vi "Fetch Measurement.vi"(6 "Enable Relative Mode (F: Disable)":bool, 7 "Combination (0: Single)":dbl(ring) items=["Single", "Feed1-Feed2", "Feed1/Feed2"], 8 "error in (no error)":errorcluster, 9 "Measurement Number (0: <0>)":i32(ring) items=["Measurement 1"=1, "Measurement 2"=2, "Measurement 3"=3, "Measurement 4"=4], 10 "Maximum Time (30000 ms)":dbl=30000.0, 11 "VISA resource name":refnum<visa-resource-name>) -> (0 "error out":errorcluster, 2 "Measurement Data (dBm or Volt)":dbl, 3 "VISA resource name out":refnum<visa-resource-name>)   [LabVIEW 2011, in "Agilent N432A.lvlib"]
doc: "Fetches the measurement data depending on the combination and relative mode settings. The combination parameter must be the same as that configured in the Configure Measurement.vi and the relative mode parameter must be the same as that configured in the Configure Relative Measurement.vi. You need to initiate an acquisition with the Initiate VI prior to calling this VI.\n\n<B>Note:</B>\n\nYou must use the Configure Measurement.vi and Configure Relative Measurement.vi to set the power meter before using this VI to fetch data.\n\nUse this VI only with other low-level VIs. The high-level VIs automatically incorporate this functionality. This VI does not check the instrument status."
uses:
  <instrlib>/Agilent N432A/Agilent N432A.lvlib
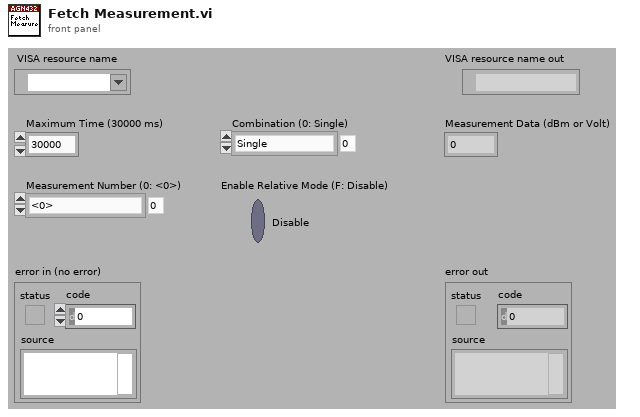
[diagram p1: front panel]
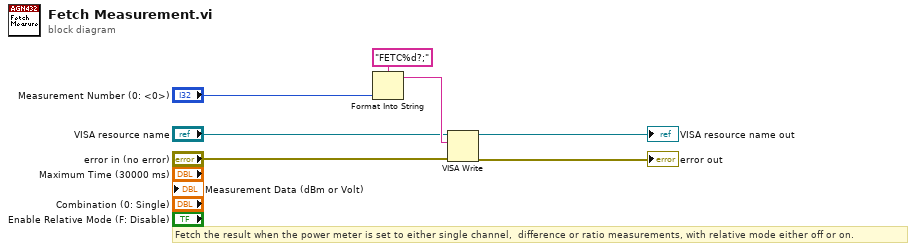
[diagram p0: block diagram]
diagram:
  # "Fetch the result when the power meter is set to either single channel,  difference or ratio measurements, with relative mode either off or on."
  n1 = Format Into String(format string="FETC%d?;", "Measurement Number (0: <0>)") -> (resulting string=w5:string)  [unwired: 2 in, 1 out]
  n2 = VISA Write(VISA resource name="VISA resource name", write buffer=w5, error in (no error)="error in (no error)") -> (VISA resource name out=→"VISA resource name out":refnum<visa-resource-name>, error out=→"error out":errorcluster)  [unwired: 1 out]
